vi "datearray_foldercreation_copyfiles_erasefiles.vi"(8 "error in":errorcluster, 11 "Cluster":T1={"path_Orig"=path "", "bo_Empty_Orig"=TRUE, "bo_exist_Orig"=TRUE, "path_Destin"=path "", "bo_Empty_Dest"=TRUE, "bo_exist_Dest"=TRUE, "bool_Erase"=FALSE, "arr_cl_lastmod_path"=[]}) -> (0 "error out":errorcluster, 3 "arr_copiedfiles":path[](array[path]))   [LabVIEW 2026]
doc: "this subVI takes the information from files founded on origin folder and \n1) checks if it is necesary create new destination folder \n2) copy file to new destination folder\n3) check if copied files are identical to origin\n4) erase original file if it is requested"
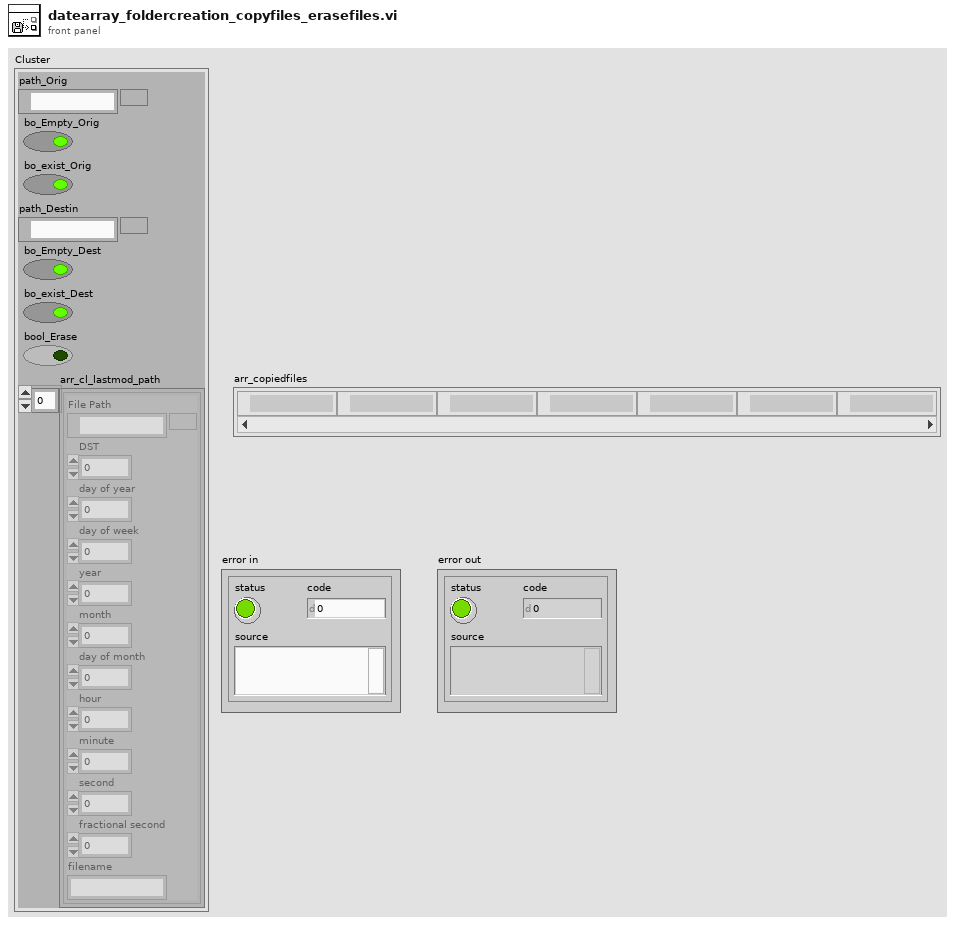
[diagram p1: front panel]
types:
  T1 = cluster{"path_Orig":path, "bo_Empty_Orig":bool, "bo_exist_Orig":bool, "path_Destin":path, "bo_Empty_Dest":bool, "bo_exist_Dest":bool, "bool_Erase":bool, "arr_cl_lastmod_path":cluster{"File Path":path, "DST":i32, "day of year":i32, "day of week":i32, "year":i32, "month":i32, "day of month":i32, "hour":i32, "minute":i32, "second":i32, "fractional second":dbl, "filename":string}[]}
  T2 = cluster{"File Path":path, "DST":i32, "day of year":i32, "day of week":i32, "year":i32, "month":i32, "day of month":i32, "hour":i32, "minute":i32, "second":i32, "fractional second":dbl, "filename":string}[]
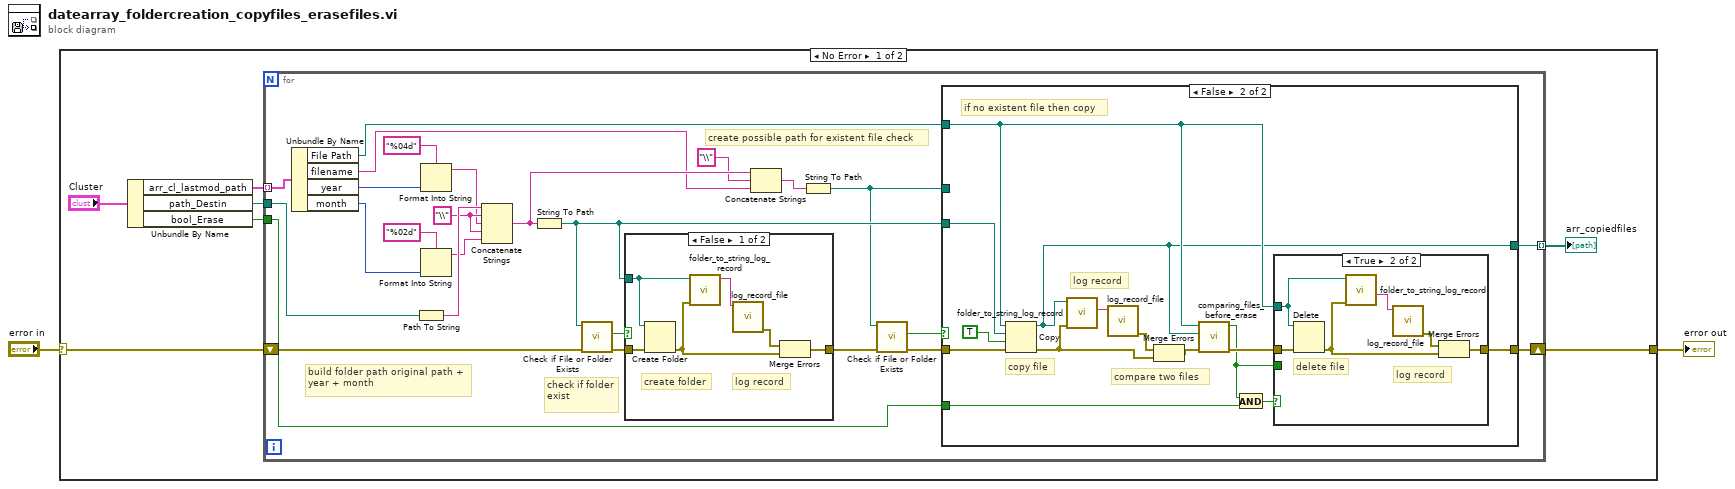
[diagram p0: block diagram]
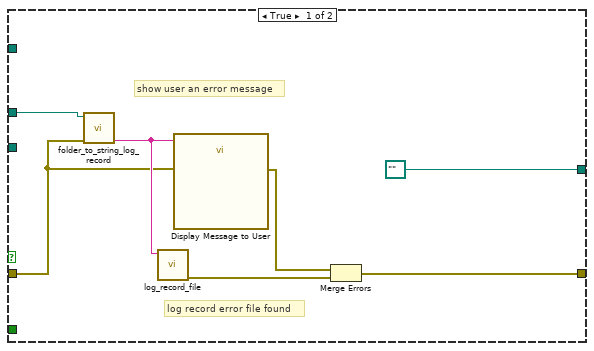
[diagram p2: hidden frame]
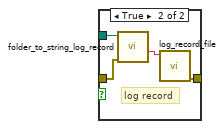
[diagram p4: hidden frame]
diagram:
  n1 = case shown="No Error" "error in" {
    selector: "error in" -> [w9 w79]
    tunnel: [w7 w79] -> w1
    frame No Error {
      n2 = Unbundle By Name("Cluster") -> ("arr_cl_lastmod_path"=w5:T2, "path_Destin"=w8:path, "bool_Erase"=w3:bool)
      n3 = for {
        tunnel: w8 -> [w34]
        tunnel: [w20] -> w6 mode=indexing
        tunnel: w5 -> [w21] mode=indexing
        tunnel: w3 -> [w16]
        shift-right: [w22] -> w7
        shift-left: w9 -> [w32]
        w33 = "\\"
        # "create possible path for existent file check"
        # "check if folder exist"
        # "build folder path original path + year + month"
        n4 = Unbundle By Name(w21) -> ("File Path"=w15:path, "filename"=w11:string, "year"=w26:i32, "month"=w29:i32)
        n5 = Path To String(path=w34) -> (string=w35:string)
        n6 = Format Into String(format string="%04d", w26) -> (resulting string=w25:string)  [unwired: 2 in, 1 out]
        n7 = Format Into String(format string="%02d", w29) -> (resulting string=w24:string)  [unwired: 2 in, 1 out]
        n8 = Concatenate Strings(w35, w33, w25, w33, w24) -> (w13:string)
        n9 = String To Path(string=w13) -> (path=w23:path)
        n10 = call <vilib>:"Check if File or Folder Exists.vi"("error in (no error)"=w32, "path"=w23) -> ("error out"=w30:errorcluster, "file or folder exists?"=w31:bool)  [unwired: 7 in, 1 out]
        n11 = case shown="False" w31 {
          tunnel: w30 -> [w77 w78]
          tunnel: [w73 w78] -> w19
          tunnel: w23 -> [w74 _]
          frame False {
            # "log record"
            # "create folder"
            n12 = Create Folder(path (use dialog)=w74, error in=w77) -> (error out=w72:errorcluster)  [unwired: 1 in, 2 out]
            n13 = call "folder_to_string_log_record.vi"("error in"=w72, "File Path"=w74) -> ("str_foldercreat"=w75:string)  [unwired: 5 in, 4 out]
            n14 = call "log_record_file.vi"("st_LogEvent"=w75) -> ("error out"=w76:errorcluster)  [unwired: 10 in]
            n15 = Merge Errors(w76, w72) -> (w73:errorcluster)
          }
          frame True {
          }
        }
        n16 = Concatenate Strings(w13, "\\", w11) -> (w14:string)
        n17 = String To Path(string=w14) -> (path=w10:path)
        n18 = call <vilib>:"Check if File or Folder Exists.vi"("error in (no error)"=w19, "path"=w10) -> ("error out"=w18:errorcluster, "file or folder exists?"=w17:bool)  [unwired: 7 in, 1 out]
        n19 = case shown="False" w17 {
          tunnel: w18 -> [w36 w56]
          tunnel: w23 -> [_ w54]
          tunnel: [w41 w53] -> w22
          tunnel: w15 -> [_ w49]
          tunnel: [path "" ("new path") w48] -> w20
          tunnel: w16 -> [_ w51]
          tunnel: w10 -> [w39 _]
          frame True {
            # "show user an error message"
            # "log record error file found"
            n20 = call "folder_to_string_log_record.vi"("error in"=w36, "File Path"=w39) -> ("str_fileerrror"=w38:string)  [unwired: 5 in, 4 out]
            n21 = call "log_record_file.vi"("st_LogEvent"=w38) -> ("error out"=w42:errorcluster)  [unwired: 10 in]
            n22 = call "Display Message to User"("error in (no error)"=w36, "Message"=w38) -> ("error out"=w40:errorcluster)  [unwired: 8 in, 1 out]
            n23 = Merge Errors(w40, w42) -> (w41:errorcluster)
          }
          frame False {
            # "compare two files"
            # "if no existent file then copy"
            # "log record"
            # "copy file"
            n24 = Copy(8:w56, 9:TRUE, 10:w54, 11:w49) -> (0:w43:errorcluster, 3:w48:path)  [unwired: 1 in, 1 out]
            n25 = call "folder_to_string_log_record.vi"("error in"=w43, "File Path"=w48) -> ("str_filecopyed"=w52:string)  [unwired: 5 in, 4 out]
            n26 = call "log_record_file.vi"("st_LogEvent"=w52) -> ("error out"=w47:errorcluster)  [unwired: 10 in]
            n27 = Merge Errors(w47, w43) -> (w44:errorcluster)
            n28 = call "comparing_files_before_erase.vi"("error in"=w44, "path_filecopied"=w48, "path_fileorigin"=w49) -> ("error out"=w46:errorcluster, "bol_equals"=w45:bool)  [unwired: 7 in]
            n29 = And(x=w45, y=w51) -> (x .and. y?=w50:bool)
            n30 = case shown="True" w50 {
              tunnel: [w58 w67] -> w53
              tunnel: w46 -> [w59 w71]
              tunnel: w49 -> [w60 w68]
              tunnel: w45 -> [w57 _]
              frame False {
                n31 = case shown="False" w57 {
                  tunnel: w60 -> [_ w65]
                  tunnel: w59 -> [w61 w62]
                  tunnel: [w61 w63] -> w58
                  frame False {
                  }
                  frame True {
                    # "log record"
                    n32 = call "folder_to_string_log_record.vi"("error in"=w62, "File Path"=w65) -> ("str_fileerased"=w64:string)  [unwired: 5 in, 4 out]
                    n33 = call "log_record_file.vi"("st_LogEvent"=w64) -> ("error out"=w63:errorcluster)  [unwired: 10 in]
                  }
                }
              }
              frame True {
                # "log record"
                # "delete file"
                n34 = Delete(path (use dialog)=w68, error in=w71) -> (error out=w66:errorcluster)  [unwired: 3 in, 2 out]
                n35 = call "folder_to_string_log_record.vi"("error in"=w66, "File Path"=w68) -> ("str_fileerased"=w69:string)  [unwired: 5 in, 4 out]
                n36 = call "log_record_file.vi"("st_LogEvent"=w69) -> ("error out"=w70:errorcluster)  [unwired: 10 in]
                n37 = Merge Errors(w70, w66) -> (w67:errorcluster)
              }
            }
          }
        }
      }
      "arr_copiedfiles" <- w6
    }
    frame Error {
    }
  }
  "error out" <- w1
